vi "GoaliePenalty.vi"(9 "Robot in":T2, 10 "balls":T5[](array[typedef])=[{"x"=-2165.869384765625, "y"=510.4085693359375, "timestamp"=timestamp(2082758857.4639893 s since 1904-01-01), "Vel_x"=0.0, "Vel_y"=0.0, "Pos Bola Est"=[]}], 11 "IA Input":T1={"our_robots"=[], "enemy_robots"=[], "balls"=[], "geometry"={"line_width"=0, "field_length"=0, "field_width"=0, "boundary_width"=0, "referee_width"=0, "goal_width"=0, "goal_depth"=0, "goal_wall_width"=0, "center_circle_radius"=0, "defense_radius"=0, "defense_stretch"=0, "free_kick_from_defense_dist"=0, "penalty_spot_from_field_line_dist"=0, "penalty_line_from_spot_dist"=0}, "IA Judge"={"stage"="", "command"="", "our_goalie_id"=0.0, "enemy_goalie_id"=0.0, "command enum"=enum."Halt", "Time"=enum."Azul"}, "Received Timestamp"=timestamp(0 s since 1904-01-01), "Events"={"Touch"=FALSE, "Ball out"=FALSE, "id touch"=0.0, "Ball out of \nVision"=FALSE, "Ball inside \nGoalie area"=FALSE, "Robot not responding"=FALSE, "Robots responding status"=[1.0, 1.0, 1.0, 1.0, 1.0, 1.0], "Enemy Ball \nPossession"=FALSE, "Pass State"=FALSE, "id end of pass"=0.0, "Kick"=FALSE, "Id ini Possession"=0.0, "Ball Possesion"=FALSE, "Id Possesion"=0.0}}) -> (2 "Robot out":T2)   [LabVIEW 2017]
uses:
  Core/AI Robot.ctl
  Functions Enum.ctl
  AttackerStates.ctl
  Core/AI Ball.ctl
  Core/AI Input.ctl
  Core/Field Size.ctl
  Core/AI Judge.ctl
  Command Enum.ctl
  Util/Events/Events.ctl
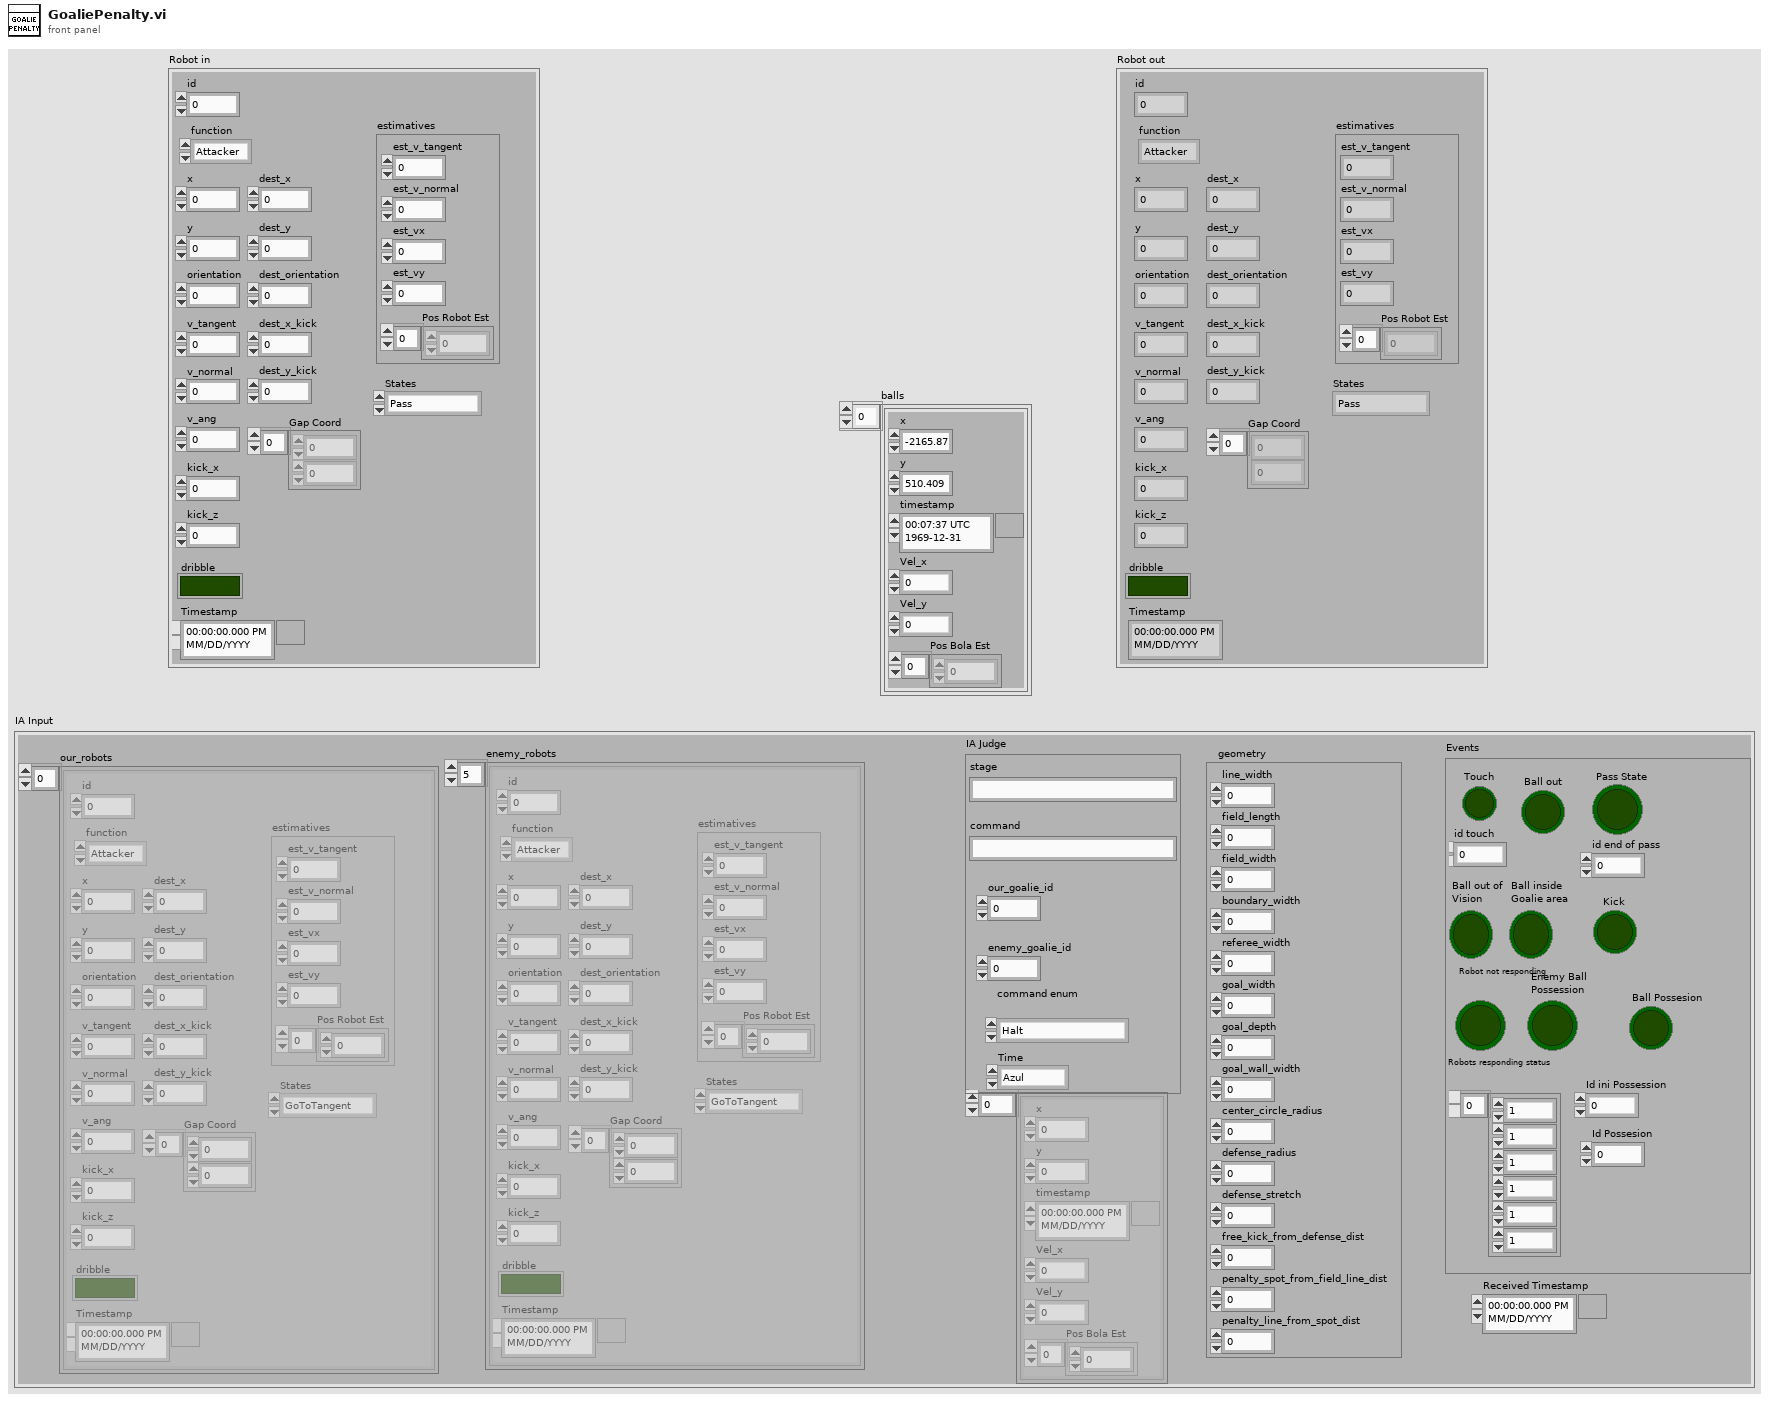
[diagram p1: front panel]
types:
  T1 = typedef "AI Input.ctl" = cluster{"our_robots":T2[], "enemy_robots":T2[], "balls":T5[], "geometry":T6, "IA Judge":T7, "Received Timestamp":timestamp, "Events":T9}
  T2 = typedef "AI Robot.ctl" = cluster{"id":u32, "function":T3, "x":dbl, "y":dbl, "orientation":dbl, "v_tangent":dbl, "v_normal":dbl, "v_ang":dbl, "kick_x":dbl, "kick_z":dbl, "dribble":bool, "Timestamp":timestamp, "dest_x":dbl, "dest_y":dbl, "dest_orientation":dbl, "estimatives":cluster{"est_v_tangent":dbl, "est_v_normal":dbl, "est_vx":dbl, "est_vy":dbl, "Pos Robot Est":dbl[]}, "dest_x_kick":dbl, "dest_y_kick":dbl, "Gap Coord":dbl[], "States":T4}
  T3 = typedef "Functions Enum.ctl" = enum16{"Attacker", "Goalie", "Defender", "Striker", "Goto 0", "Dummy", "Kicker", "ZigZag"}
  T4 = typedef "AttackerStates.ctl" = enum16{"Pass", "GoToTangent", "BallGetting", "GoToKick", ""}
  T5 = typedef "AI Ball.ctl" = cluster{"x":dbl, "y":dbl, "timestamp":timestamp, "Vel_x":dbl, "Vel_y":dbl, "Pos Bola Est":dbl[]}
  T6 = typedef "Field Size.ctl" = cluster{"line_width":u32, "field_length":u32, "field_width":u32, "boundary_width":u32, "referee_width":u32, "goal_width":u32, "goal_depth":u32, "goal_wall_width":u32, "center_circle_radius":u32, "defense_radius":u32, "defense_stretch":u32, "free_kick_from_defense_dist":u32, "penalty_spot_from_field_line_dist":u32, "penalty_line_from_spot_dist":u32}
  T7 = typedef "AI Judge.ctl" = cluster{"stage":string, "command":string, "our_goalie_id":dbl, "enemy_goalie_id":dbl, "command enum":T8, "Time":enum16{"Azul", "Amarelo"}}
  T8 = typedef "Command Enum.ctl" = enum16{"Halt", "Stop", "Force Start", "PKA Normal Start", "Prepare Kickoff Ally", "PKE Normal Start", "Prepare Kickoff Enemy", "Prepare Penalty Ally", "PPA Normal Start", "Prepare Penalty Enemy", "PPE Normal Start", "Direct Free Enemy", "Direct Free Ally", "Indirect Free Enemy", "Indirect Free Ally", "Timeout Enemy", "Timeout Ally", "Goal Enemy", "Goal Ally", "Ball Placement Enemy", "Ball Placement Ally", "Normal Half Time", "Extra Time Break", "Extra Half Time", "None", "Post Game"}
  T9 = typedef "Events.ctl" = cluster{"Touch":bool, "Ball out":bool, "id touch":dbl, "Ball out of \nVision":bool, "Ball inside \nGoalie area":bool, "Robot not responding":bool, "Robots responding status":dbl[], "Enemy Ball \nPossession":bool, "Pass State":bool, "id end of pass":dbl, "Kick":bool, "Id ini Possession":dbl, "Ball Possesion":bool, "Id Possesion":dbl}
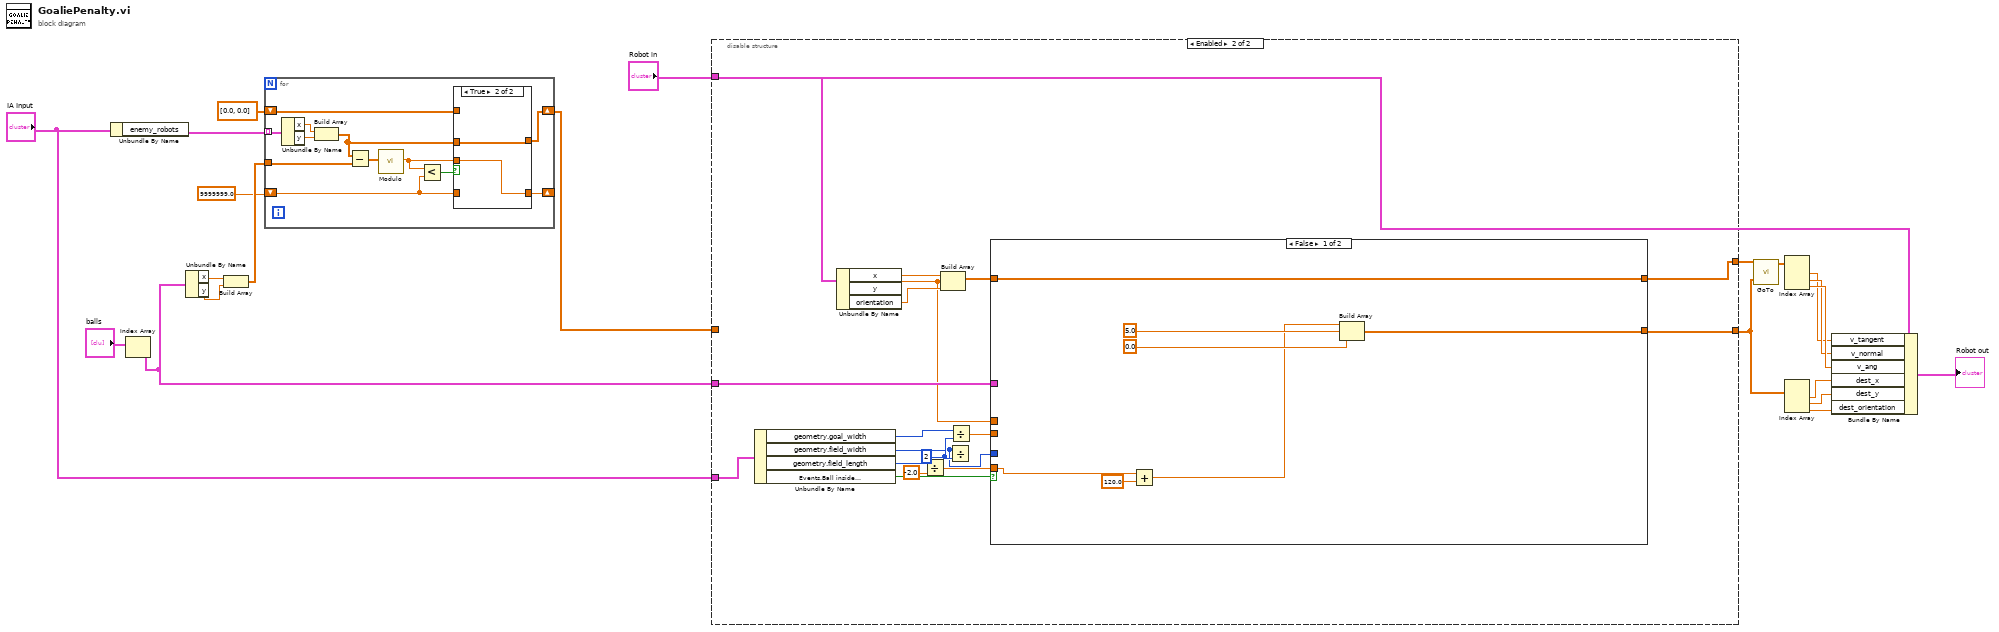
[diagram p0: block diagram]
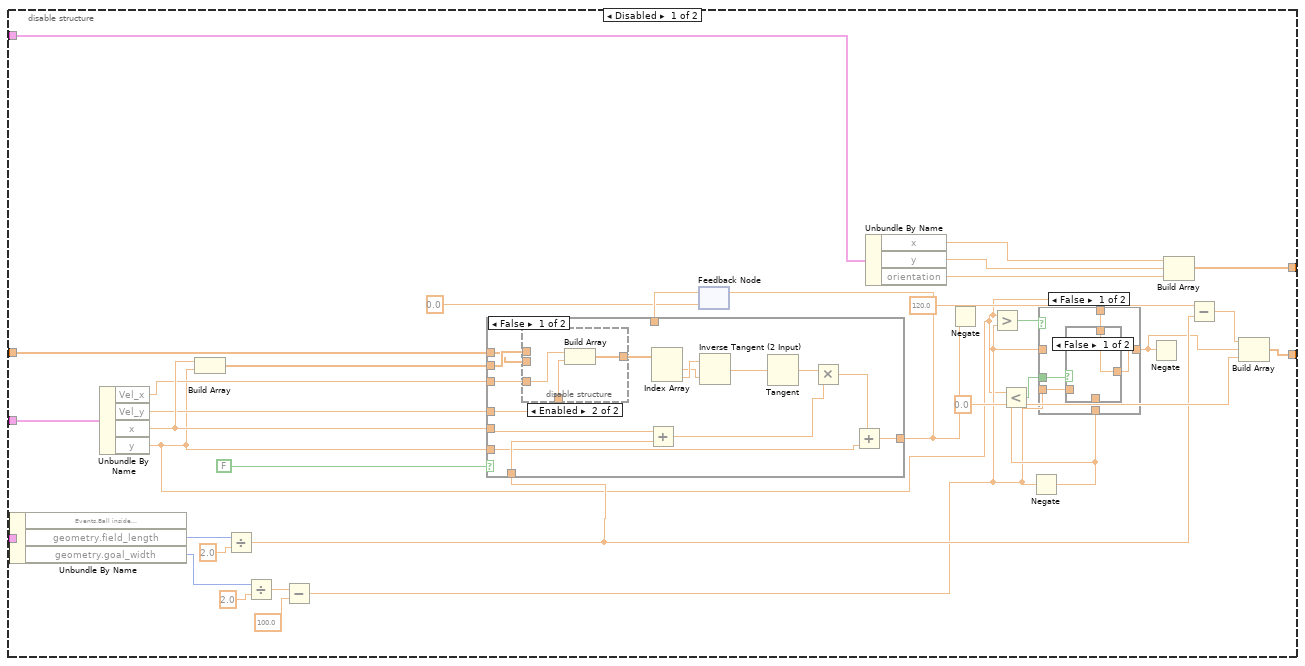
[diagram p2: hidden frame]
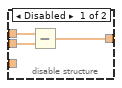
[diagram p5: hidden frame]
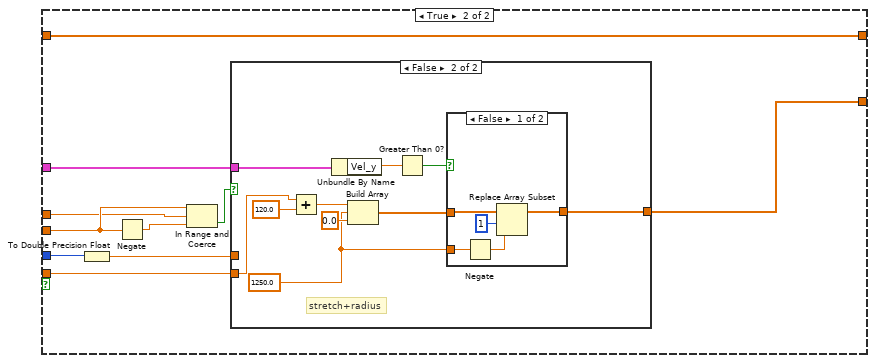
[diagram p7: hidden frame]
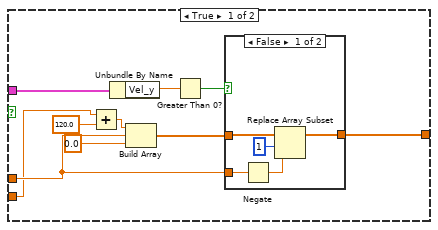
[diagram p8: hidden frame]
diagram:
  n1 = Unbundle By Name("IA Input") -> ("enemy_robots"=w9:T2[])
  n2 = Index Array(array="balls") -> (element=w8:T5)  [unwired: 1 in]
  n3 = Unbundle By Name(w8) -> ("x"=w7:dbl, "y"=w6:dbl)
  n4 = Build Array(w7, w6) -> (w5:dbl[])
  n5 = for {
    tunnel: w9 -> [w33] mode=indexing
    tunnel: w5 -> [w30]
    shift-right: [w24] -> _
    shift-left: 9999999.0 -> [w28]
    shift-right: [w25] -> w1
    shift-left: dbl[] [0.0, 0.0] -> [w22]
    n6 = Unbundle By Name(w33) -> ("x"=w32:dbl, "y"=w31:dbl)
    n7 = Build Array(w32, w31) -> (w26:dbl[])
    n8 = Subtract(x=w26, y=w30) -> (x-y=w29:dbl[])
    n9 = call "Modulo.vi"("2D vector"=w29) -> ("Modulo"=w23:dbl)  [unwired: 10 in]
    n10 = Less?(x=w23, y=w28) -> (x < y?=w27:bool)
    n11 = case shown="True" w27 {
      tunnel: w28 -> [w34 _]
      tunnel: [w35 w37] -> w25
      tunnel: w26 -> [_ w37]
      tunnel: [w34 w36] -> w24
      tunnel: w23 -> [_ w36]
      tunnel: w22 -> [w35 _]
      frame False {
      }
      frame True {
      }
    }
  }
  n12 = disable-structure shown="Enabled" {
    disable-tunnel: [w70 w113] -> w15
    disable-tunnel: "Robot in" -> [w68 w115]
    disable-tunnel: [w66 w107] -> w10
    disable-tunnel: w8 -> [w64 w106]
    disable-tunnel: "IA Input" -> [w62 w117]
    disable-tunnel: w1 -> [w57 _]
    frame Disabled {
      n13 = Unbundle By Name(w62) -> ("geometry.field_length"=w61:u32, "geometry.goal_width"=w49:u32)  [unwired: 1 out]
      n14 = Unbundle By Name(w64) -> ("Vel_x"=w44:dbl, "Vel_y"=w43:dbl, "x"=w59:dbl, "y"=w39:dbl)
      n15 = Build Array(w59, w39) -> (w58:dbl[])
      n16 = Divide(x=w61, y=2.0) -> (x/y=w52:dbl)
      n17 = Divide(x=w49, y=2.0) -> (x/y=w42:dbl)
      n18 = Subtract(x=w42, y=100.0) -> (x-y=w41:dbl)
      n19 = feedback #1(0.0) -> (w56:dbl)
      n20 = case shown="False" FALSE {
        tunnel: w39 -> [w85 _]
        tunnel: w59 -> [w83 _]
        tunnel: w52 -> [w93 _]
        tunnel: w58 -> [w92 _]
        tunnel: w57 -> [w91 _]
        tunnel: [w84 w100] -> w51
        tunnel: w56 -> [_ w100]
        tunnel: w44 -> [w80 _]
        tunnel: w43 -> [w79 _]
        frame False {
          n21 = disable-structure shown="Enabled" {
            disable-tunnel: w92 -> [w96 _]
            disable-tunnel: w91 -> [w95 _]
            disable-tunnel: [w94 w97] -> w90
            disable-tunnel: w80 -> [_ w99]
            disable-tunnel: w79 -> [_ w98]
            frame Disabled {
              n22 = Subtract(x=w96, y=w95) -> (x-y=w94:dbl[])
            }
            frame Enabled {
              n23 = Build Array(w99, w98) -> (w97:dbl[])
            }
          }
          n24 = Add(x=w83, y=w93) -> (x+y=w87:dbl)
          n25 = Index Array(array=w90) -> (element #1=w88:dbl, element #2=w89:dbl)  [unwired: 2 in]
          n26 = Inverse Tangent (2 Input)(1:w88, 2:w89) -> (0:w81:dbl)
          n27 = Tangent(1:w81) -> (0:w82:dbl)
          n28 = Multiply(x=w82, y=w87) -> (x*y=w86:dbl)
          n29 = Add(x=w86, y=w85) -> (x+y=w84:dbl)
        }
        frame True {
        }
      }
      n30 = feedback-in #1(w51) -> ()
      n31 = Unbundle By Name(w68) -> ("x"=w65:dbl, "y"=w67:dbl, "orientation"=w69:dbl)
      n32 = Negate(x=w51) -> ()  [unwired: 1 out]
      n33 = Greater?(x=w39, y=w41) -> (0:w48:bool)
      n34 = Negate(x=w41) -> (-x=w46:dbl)
      n35 = Less?(x=w39, y=w46) -> (x < y?=w47:bool)
      n36 = case shown="False" w48 {
        tunnel: w41 -> [w75 _]
        tunnel: [w74 w78] -> w38
        tunnel: w47 -> [w73 _]
        tunnel: w41 -> [_ w78]
        tunnel: w46 -> [w72 _]
        tunnel: w39 -> [w71 _]
        frame False {
          n37 = case shown="False" w73 {
            tunnel: [w76 w77] -> w74
            tunnel: w75 -> [_ _]
            tunnel: w72 -> [_ w77]
            tunnel: w71 -> [w76 _]
            frame False {
            }
            frame True {
            }
          }
        }
        frame True {
        }
      }
      n38 = Negate(x=w38) -> ()  [unwired: 1 out]
      n39 = Build Array(w65, w67, w69) -> (w70:dbl[])
      n40 = Subtract(x=120.0 ("element"), y=w52) -> (x-y=w53:dbl)
      n41 = Build Array(w53, w38, 0.0 ("element")) -> (w66:dbl[])
    }
    frame Enabled {
      w105 = u32 2 ("y")
      n42 = Unbundle By Name(w117) -> ("geometry.goal_width"=w104:u32, "geometry.field_width"=w101:u32, "geometry.field_length"=w110:u32, "Events.Ball inside \nGoalie area"=w116:bool)
      n43 = Unbundle By Name(w115) -> ("x"=w114:dbl, "y"=w102:dbl, "orientation"=w111:dbl)
      n44 = Divide(x=w110, y=-2.0) -> (x/y=w108:dbl)
      n45 = Build Array(w114, w102, w111) -> (w112:dbl[])
      n46 = Divide(x=w101, y=w105) -> ()  [unwired: 1 out]
      n47 = Divide(x=w104, y=w105) -> (x/y=w103:dbl)
      n48 = case shown="False" w116 {
        tunnel: [w124 w133] -> w113
        tunnel: w112 -> [w124 w133]
        tunnel: w108 -> [w120 w127]
        tunnel: [w121 w132] -> w107
        tunnel: w106 -> [_ w134]
        tunnel: w101 -> [_ w126]
        tunnel: w103 -> [_ w129]
        tunnel: w102 -> [_ w128]
        frame False {
          n49 = Add(x=w120, y=120.0) -> (x+y=w119:dbl)
          n50 = Build Array(w119, 5.0 ("element"), 0.0 ("element")) -> (w121:dbl[])
        }
        frame True {
          n51 = To Double Precision Float(number=w126) -> (double precision float=w125:dbl)
          n52 = Negate(x=w129) -> (-x=w130:dbl)
          n53 = In Range and Coerce(upper limit=w129, x=w128, lower limit=w130) -> (In Range?=w131:bool)  [unwired: 1 out]
          n54 = case shown="False" w131 {
            tunnel: w134 -> [w144 w160]
            tunnel: w125 -> [w139 _]
            tunnel: [w138 w155] -> w132
            tunnel: w127 -> [w135 w151]
            frame True {
              n55 = Add(x=w135, y=120.0) -> (x+y=w136:dbl)
              n56 = Unbundle By Name(w144) -> ("Vel_y"=w142:dbl)
              n57 = Build Array(w136, w139, 0.0 ("element")) -> (w140:dbl[])
              n58 = Greater Than 0?(x=w142) -> (x > 0?=w143:bool)
              n59 = case shown="False" w143 {
                tunnel: w140 -> [w149 w150]
                tunnel: w139 -> [w147 _]
                tunnel: [w145 w150] -> w138
                frame False {
                  n60 = Negate(x=w147) -> (-x=w146:dbl)
                  n61 = Replace Array Subset(array=w149, new element=w146, index=1) -> (w145:dbl[])
                }
                frame True {
                }
              }
            }
            frame False {
              w154 = 1250.0
              # "stretch+radius"
              n62 = Add(x=w151, y=120.0) -> (x+y=w152:dbl)
              n63 = Unbundle By Name(w160) -> ("Vel_y"=w158:dbl)
              n64 = Build Array(w152, w154, 0.0 ("element")) -> (w156:dbl[])
              n65 = Greater Than 0?(x=w158) -> (x > 0?=w159:bool)
              n66 = case shown="False" w159 {
                tunnel: w156 -> [w165 w166]
                tunnel: w154 -> [w163 _]
                tunnel: [w161 w166] -> w155
                frame False {
                  n67 = Negate(x=w163) -> (-x=w162:dbl)
                  n68 = Replace Array Subset(array=w165, new element=w162, index=1) -> (w161:dbl[])
                }
                frame True {
                }
              }
            }
          }
        }
      }
    }
  }
  n69 = call "GoTo.vi"("Target"=w10, "Position"=w15) -> ("Output\nVelocity"=w14:dbl[])  [unwired: 8 in, 1 out]
  n70 = Index Array(array=w14) -> (element #1=w19:dbl, element #2=w20:dbl, element #3=w21:dbl)  [unwired: 3 in]
  n71 = Index Array(array=w10) -> (element #1=w16:dbl, element #2=w17:dbl, element #3=w18:dbl)  [unwired: 3 in]
  n72 = Bundle By Name(cluster="Robot in", "v_tangent"=w19, "v_normal"=w20, "v_ang"=w21, "dest_x"=w16, "dest_y"=w17, "dest_orientation"=w18) -> (→"Robot out":T2)
